vi "FXP NILIA_MovingAverage.vi"(6 "decimate":i16=1024, 9 "stages":i8=1, 11 "input":i64) -> (3 "output":i64)   [LabVIEW 2012]
uses:
  <vilib>/Platform/TimedLoop/XDataNode/timing_clust.ctl
  <vilib>/Platform/TimedLoop/XDataNode/nitl_modes.ctl
  <vilib>/Platform/TimedLoop/XDataNode/wakeup.ctl
  <vilib>/rvi/DataTransferAndStorage/Container/Common/niFpgaContainerMetaDataKey.ctl
  <vilib>/rvi/DataTransferAndStorage/Container/Common/niFpgaContainerState.ctl
  <vilib>/rvi/DataTransferAndStorage/Container/Common/niFpgaDataTypeControl.ctl
  <vilib>/rvi/DataTransferAndStorage/Container/Common/niFpgaContainerImplementationControl.ctl
  <vilib>/rvi/DataTransferAndStorage/Container/Common/niFpgaContainerArbitrationOptionsControl.ctl
  <vilib>/rvi/DataTransferAndStorage/Container/Common/niFpgaTransferTypeControl.ctl
  <vilib>/rvi/DataTransferAndStorage/Container/Common/niFpgaContainerInitializationParameters.ctl
  <vilib>/rvi/Memory/Memory_Types/niFpgaMemoryInterfaceConfiguration.ctl
  <vilib>/rvi/FIFO/Fifo_Types/niFpgaFifoControlLogicControl.ctl
  <vilib>/rvi/DataTransferAndStorage/Container/Common/niFpgaContainerGetUniqueNameForEmu.vi
  <vilib>/rvi/DataTransferAndStorage/Container/Common/niFpgaContainerSetEmuInfo.vi
  <vilib>/rvi/eio/common/nirviEmuReportErrorAndStop.vi
  <vilib>/rvi/Emulation/niFpgaSctlEmulationRegisterWithScheduler.vi
  <vilib>/rvi/Memory/Memory_Emulation/niFpgaMemoryEmulationCacheClearOnFirstRun.vi
  <vilib>/rvi/Memory/Memory_Emulation/nirvimemoryEmulationManagerCache_MakeExclusive.vi
  <vilib>/rvi/Memory/Memory_Emulation/niFpgaMemoryEmulationValidateCache.vi
  <vilib>/rvi/Memory/Memory_Emulation/nirvimemoryEmulationManagerCache_ReleaseExclusive.vi
  <vilib>/rvi/Memory/Memory_Emulation/nirvimemoryEmulationManagerCache_InsertValue.vi
  <vilib>/Utility/error.llb/Clear Errors.vi
  <vilib>/rvi/Memory/Memory_Emulation/nirvimemoryEmulationManagerCache_GetValue.vi
  <vilib>/rvi/Memory/Memory_Emulation/nirvimemoryEmulationManagerCache_SetValue.vi
  <vilib>/rvi/Emulation/niFpgaSctlEmulationResourceMgr.vi
  <vilib>/rvi/Emulation/niFpgaSctlEmulationScheduler.vi
  <vilib>/Platform/TimedLoop/XDataNode/XDataNode.xnode
  <vilib>/rvi/LocalResourceManager/LocalResourceManager.xnode
  <vilib>/rvi/FXPMathLib/basic elements/FxpDiscreteDelay/XNode/nifxpmath_DiscreteDelay.xnode
  <vilib>/rvi/DataTransferAndStorage/Container/XNode/niFpgaContainer.xnode
  <vilib>/rvi/Memory/Memory_Emulation/nirvimemoryEmulation.vi
  <vilib>/Platform/TimedLoop/XDataNode/XDNodeRunTimeDep.lvlib
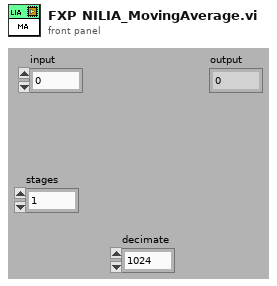
[diagram p1: front panel]
types:
  T1 = typedef "XDNodeRunTimeDep.lvlib/timing_clust.ctl" = cluster{"Expected End [f-1]":u64, "Actual End [f-1]":u64, "Finished Late? [f-1]":bool, "Expected End [i-1]":u64, "Actual End [i-1]":u64, "Finished Late? [i-1]":bool, "Expected Start [i]":u64, "Actual Start [i]":u64, "Expected Start [f]":u64, "Actual Start [f]":u64, "Source Name":string, "Structure Name":string, "Period":i64, "Deadline":i64, "Offset":i64, "Start":i64, "Priority":i32, "Timeout":i32, "Mode":T2, "Wakeup Reason":T3, "Error":errorcluster, "Source Type":string, "Secondary Source Type":string, "Global End Time":u64, "Global Start Time":u64, "Frame Duration":u64, "Iteration Duration":u64, "Assigned CPU":i32, "I/O Scan Engine Mode":u32}
  T2 = typedef "XDNodeRunTimeDep.lvlib/nitl_modes.ctl" = enum32{"No Change", "Process missed periods, maintain original phase", "Discard missed periods, maintain original phase", "Process missed periods, ignore original phase", "Discard missed periods, ignore original phase"}
  T3 = typedef "XDNodeRunTimeDep.lvlib/wakeup.ctl" = enum32{"Normal", "Aborted", "Asynchronous wakeup", "Timing source error", "Timed loop error", "Timeout"}
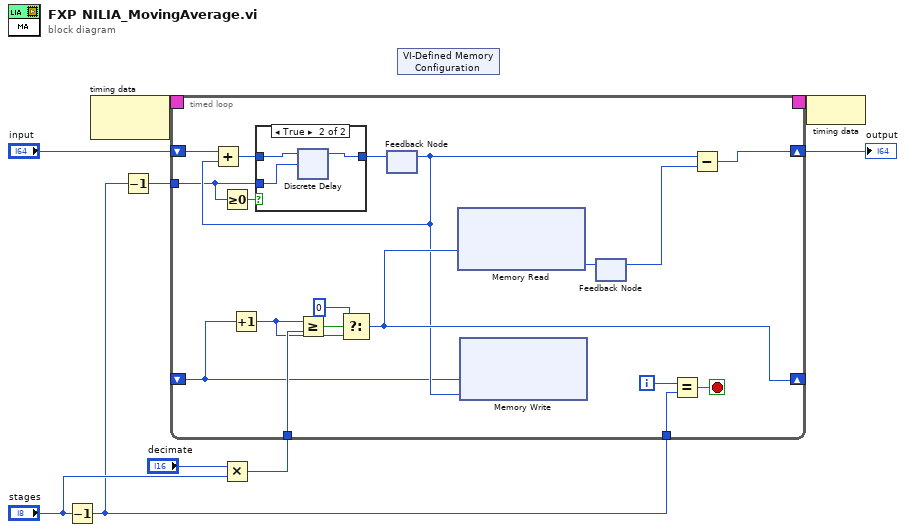
[diagram p0: block diagram]
diagram:
  n1 = Decrement(x="stages") -> (x-1=w2:i8)
  n2 = node-c288() -> (w9:T1)  [unwired: 1 in]
  n3 = Decrement(x=w2) -> (x-1=w1:i8)
  n4 = Multiply(x="decimate", y="stages") -> (x*y=w3:i16)
  n5 = timed-loop {
    timing: w9 -> [_]
    timing-out: [_] -> w8
    shift-right: [w25] -> w6
    shift-left: "input" -> [w27]
    shift-right: [w17] -> _
    shift-left: _ -> [w11]
    tunnel: w2 -> [w21]
    tunnel: w3 -> [w20]
    tunnel: w1 -> [w12]
    i -> [w24]
    stop <- w23 stop-if-true
    n6 = Greater Or Equal To 0?(x=w12) -> (x >= 0?=w13:bool)
    n7 = Increment(x=w11) -> (x+1=w10:i16)
    n8 = Greater Or Equal?(x=w10, y=w20) -> (x >= y?=w19:bool)
    n9 = Select(t=i16 0, s=w19, f=w10) -> (s? t:f=w17:i16)
    n10 = feedback #1() -> (w16:i64)  [unwired: 1 in]
    n11 = Add(x=w27, y=w16) -> (x+y=w15:i64)
    n12 = case shown="True" w13 {
      tunnel: w15 -> [w28 w31]
      tunnel: [w28 w30] -> w14
      tunnel: w12 -> [_ w29]
      frame False {
      }
      frame True {
        n13 = xnode "Discrete Delay"("D"=w31, "n-1[0..15]"=w29) -> ("Q"=w30:i64)
      }
    }
    n14 = feedback-in #1(w14) -> ()
    n15 = xnode ("Memory Read")("Address"=w17) -> ("Data"=w26:i64)  [unwired: 1 in, 1 out]
    n16 = xnode ("Memory Write")("Address"=w11, "Data"=w16) -> ()  [unwired: 1 in, 1 out]
    n17 = feedback-in #2(w26) -> ()
    n18 = feedback #2() -> (w22:i64)  [unwired: 1 in]
    n19 = Equal?(x=w24, y=w21) -> (x = y?=w23:bool)
    n20 = Subtract(x=w16, y=w22) -> (x-y=w25:i64)
  }
  "output" <- w6
  n21 = xnode "VI-Defined Memory Configuration"() -> ()  [unwired: 1 out]
  n22 = node-c288(w8) -> ()
